vi "Get Field.vi"(6 "Axis":T1, 8 "error in (no error)":errorcluster, 11 "Instrument.VRM in":refnum<class "Instrument.OxfordVRM.lvclass">) -> (0 "error out":errorcluster, 2 "Field (T)":dbl[](array[numeric]), 3 "Instrument.VRM out":refnum<class "Instrument.OxfordVRM.lvclass">)   [LabVIEW 2019, in "Instrument.OxfordVRM.lvclass"]
uses:
  Instrument.OxfordVRM.lvclass
  C:/Program Files (x86)/National Instruments/LabVIEW 2019/user.lib/LevyLab/Levylab Instruments/SMOs/Instrument/Instrument.lvclass
  Typedefs/VRM Magnet Axis--Enum.ctl
  Typedefs/Instrument.VRM.Commands-enum.ctl
  <userlib>/LevyLab/Instrument Framework/SMOs/Instrument/Instrument.lvclass/Instrument.ctl
  28e49aab-af7c-4390-a0d4-9e6a818264a5.vi
  28e49aab-af7c-4390-a0d4-9e6a818264a5.vi/c3adec56-f445-4f56-a77a-1ba4ece32de5.vi
  28e49aab-af7c-4390-a0d4-9e6a818264a5.vi/c3adec56-f445-4f56-a77a-1ba4ece32de5.vi/8a5e7313-1f17-4e4c-bbb7-eca125fd123a.vi
  <userlib>/LevyLab/Instrument Framework/SMOs/Instrument/API/Send and Receive.vi
  28e49aab-af7c-4390-a0d4-9e6a818264a5.vi/c3adec56-f445-4f56-a77a-1ba4ece32de5.vi/8a5e7313-1f17-4e4c-bbb7-eca125fd123a.vi/4473e125-ab3e-4b17-84e1-57644d00459e.vi
  28e49aab-af7c-4390-a0d4-9e6a818264a5.vi/c3adec56-f445-4f56-a77a-1ba4ece32de5.vi/8a5e7313-1f17-4e4c-bbb7-eca125fd123a.vi/dbc2f059-4560-4f86-b5b4-f2ac57237942.vi
  <userlib>/LevyLab/Instrument Framework/SMOs/Instrument/API/Enum to String.vi
  <userlib>/LevyLab/Instrument Framework/SMOs/RemoteControl/API/Send and Receive.vi
  <vilib>/Utility/Data Type/Get Type Information.vi
  <vilib>/JDP Science/JSONtext/JSON text to Variant.vi
  <vilib>/JDP Science/JSONtext/LVClass Serializer/JSONtext LVClass Serializer.lvclass
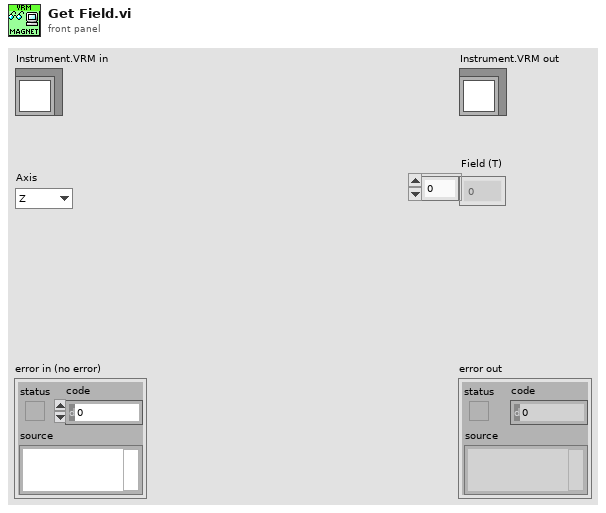
[diagram p1: front panel]
types:
  T1 = typedef "Instrument.OxfordVRM.lvclass/VRM Magnet Axis--Enum.ctl" = enum16{"Z", "X", "Y", "ALL"}
  T2 = typedef "Instrument.OxfordVRM.lvclass/Instrument.VRM.Commands-enum.ctl" = enum16{"setAction", "setTarget", "setMagnetField", "getStatus", "getTarget", "getMagnetField"}
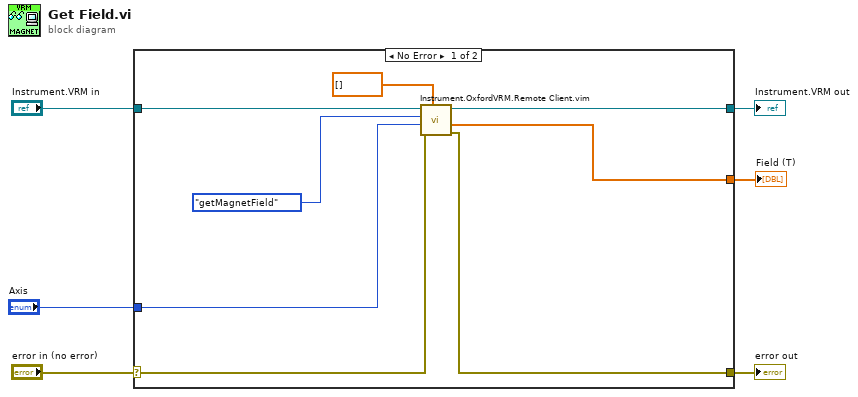
[diagram p0: block diagram]
diagram:
  n1 = case shown="No Error" "error in (no error)" {
    selector: "error in (no error)" -> [w13 w16]
    tunnel: [w11 w16] -> w5
    tunnel: "Instrument.VRM in" -> [w10 w15]
    tunnel: [w12 _] -> w3
    tunnel: [w9 w15] -> w2
    tunnel: "Axis" -> [w8 _]
    frame No Error {
      n2 = call "Instrument.OxfordVRM.Remote Client.vim"("Data Out type"=dbl[] [], "error in (no error)"=w13, "Data"=w8, "Commands"=Instrument.VRM.Commands-enum."getMagnetField", "Instrument.VRM in"=w10) -> ("error out"=w11:errorcluster, "Data out"=w12:dbl[], "Instrument.VRM out"=w9:refnum<class "Instrument.OxfordVRM.lvclass">)  [unwired: 4 in]
    }
    frame Error {
    }
  }
  "error out" <- w5
  "Instrument.VRM out" <- w2
  "Field (T)" <- w3
